vi "Get Ungoaled Categories.vi"(8 "error in (no error)":errorcluster, 9 "Month":T1, 10 "YYYY":i32, 11 "Database in":refnum<class "Account History.lvclass">) -> (0 "error out":errorcluster, 2 "Categories with No Goal":refnum<class "Category.lvclass">[](array[class]), 3 "Database out":refnum<class "Account History.lvclass">)   [LabVIEW 2018, in "Account History.lvclass"]
uses:
  Account History.lvclass
  Category/Category.lvclass
  Month.ctl
  WhichMonth/WhichMonth.lvclass
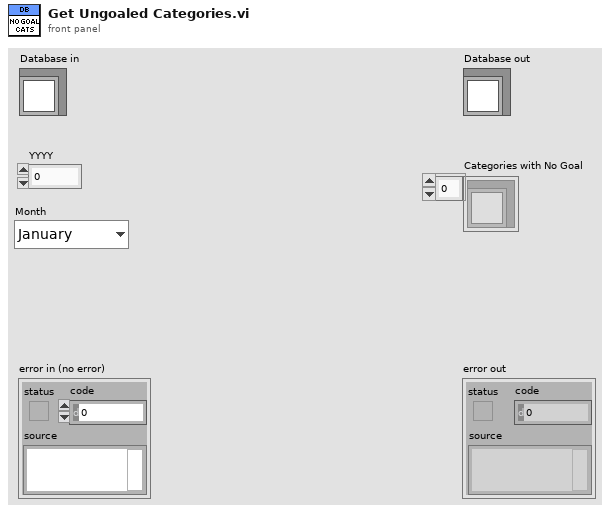
[diagram p1: front panel]
types:
  T1 = typedef "WhichMonth.lvclass/Month.ctl" = enum16{"January", "February", "March", "April", "May", "June", "July", "August", "September", "October", "November", "December"}
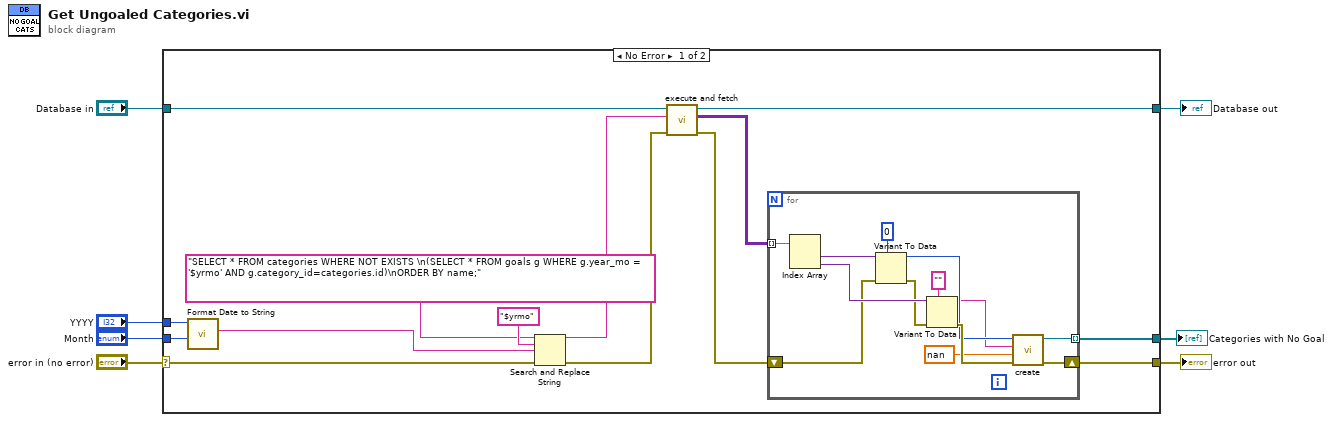
[diagram p0: block diagram]
diagram:
  n1 = case shown="No Error" "error in (no error)" {
    selector: "error in (no error)" -> [w20 w36]
    tunnel: [w14 w36] -> w6
    tunnel: [w15 w35] -> w4
    tunnel: "Database in" -> [w12 w35]
    tunnel: [w13 _] -> w3
    tunnel: "YYYY" -> [w10 _]
    tunnel: "Month" -> [w9 _]
    frame No Error {
      n2 = call "Format Date to String.vi"("Month"=w9, "YYYY"=w10) -> ("Year-Mo"=w8:string)  [unwired: 9 in]
      n3 = Search and Replace String(input string="SELECT * FROM categories WHERE NOT EXISTS \n(SELECT * FROM goals g WHERE g.year_mo = '$yrmo' AND g.category_id=categories.id)\nORDER BY name;", search string="$yrmo", replace string=w8, error in=w20) -> (result string=w16:string, error out=w17:errorcluster)  [unwired: 4 in, 2 out]
      n4 = call "execute and fetch.vi"("error in (no error)"=w17, "SQL query"=w16, "Database in"=w12) -> ("error out"=w18:errorcluster, "recordset data"=w19:variant[][], "Database out"=w15:refnum<class "Account History.lvclass">)  [unwired: 5 in, 1 out]
      n5 = for {
        tunnel: w19 -> [w27] mode=indexing
        shift-right: [w33] -> w14
        shift-left: w18 -> [w26]
        tunnel: [w34] -> w13 mode=indexing
        n6 = Index Array(array=w27) -> (element #1=w32:variant, element #2=w31:variant)  [unwired: 2 in]
        n7 = Variant To Data(error in=w26, type=0, Variant=w32) -> (data=w24:i32, error out=w28:errorcluster)
        n8 = Variant To Data(error in=w28, type="", Variant=w31) -> (data=w23:string, error out=w25:errorcluster)
        n9 = call "create.vi"("error in (no error)"=w25, 9:nan ("Default Goal Amount"), "Default Goal Amount"=w23, "Name"=w24) -> ("error out"=w33:errorcluster, "Category out"=w34:refnum<class "Category.lvclass">)  [unwired: 6 in]
      }
    }
    frame Error {
    }
  }
  "error out" <- w6
  "Database out" <- w4
  "Categories with No Goal" <- w3
